vi "Write Limit Current.vi"(8 "error in":errorcluster, 10 "OverCurrent_Protect":dbl, 11 "SimulatedPS in":refnum<class "SimulatedPS.lvclass">) -> (0 "error out":errorcluster, 3 "SimulatedPS out":refnum<class "SimulatedPS.lvclass">)   [LabVIEW 2019, in "SimulatedPS.lvlib" / "SimulatedPS.lvclass"]
uses:
  Library/SimulatedPS.lvclass
  builds/Instruments/PowerSupply.lvlibp/Library/PowerSupply.lvclass
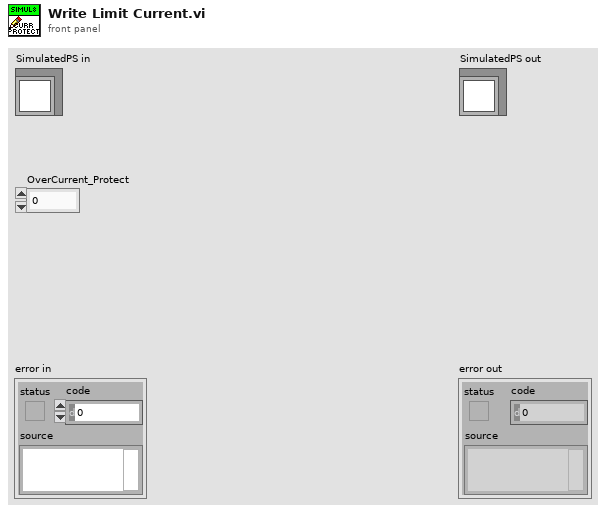
[diagram p1: front panel]
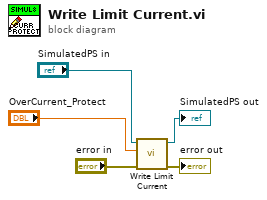
[diagram p0: block diagram]
diagram:
  n1 = call-parent "Write Limit Current.vi"("error in"="error in", "OverCurrent_Protect"="OverCurrent_Protect", "PowerSupply in"="SimulatedPS in") -> ("error out"=→"error out":errorcluster, "PowerSupply out"=→"SimulatedPS out":refnum<class "SimulatedPS.lvclass">)  [unwired: 7 in]
